vi "Boiler Controller.vi"(8 "error in":errorcluster, 9 "Controller Configuration":T1, 10 "Notifiers":T2, 11 "Message Queues":T3) -> (0 "error out":errorcluster)   [LabVIEW 2014, in "Controller.lvlib"]
uses:
  Controller.lvlib
  support/Message Queue/All Message Queues.ctl
  support/Message Queue/Message Cluster.ctl
  support/Notifiers/Notifiers.ctl
  Controller Configuration.ctl
  controls/MHL UI Data.ctl
  controls/MHL Status.ctl
  support/Boiler System Globals.vi
  <vilib>/Utility/error.llb/Error Cluster From Error Code.vi
  <vilib>/ErrorRing/Error Ring.xnode
  support/Message Queue/Message Queue.lvlib
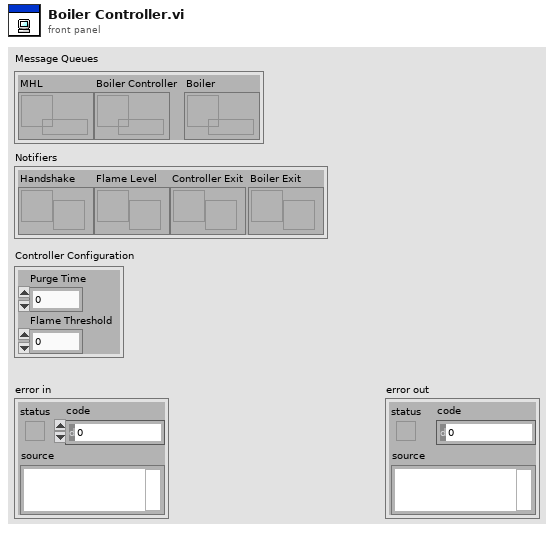
[diagram p1: front panel]
types:
  T1 = typedef "Controller.lvlib/Controller Configuration.ctl" = cluster{"Purge Time":u32, "Flame Threshold":u32}
  T2 = typedef "Notifiers.ctl" = cluster{"Handshake":refnum<notifier>, "Flame Level":refnum<notifier>, "Controller Exit":refnum<notifier>, "Boiler Exit":refnum<notifier>}
  T3 = typedef "Message Queue.lvlib/All Message Queues.ctl" = cluster{"MHL":refnum<queue>, "Boiler Controller":refnum<queue>, "Boiler":refnum<queue>}
  T4 = enum16{"open", "replace", "create", "open or create", "replace or create", "replace or create with confirmation"}
  T5 = typedef "MHL Status.ctl" = enum16{"Lockout", "Ready", "Pre-Purge", "Pre-Purge Complete", "Pilot On", "Boiler Running", "Shutdown", "Purge"}
  T6 = typedef "MHL UI Data.ctl" = cluster{"Status":string, "Fuel Control Valve":u32, "Primary Fan":bool, "Pilot Gas Valve":bool, "Pilot":bool, "Forced Draft Fan":bool, "MHL Status":T5}
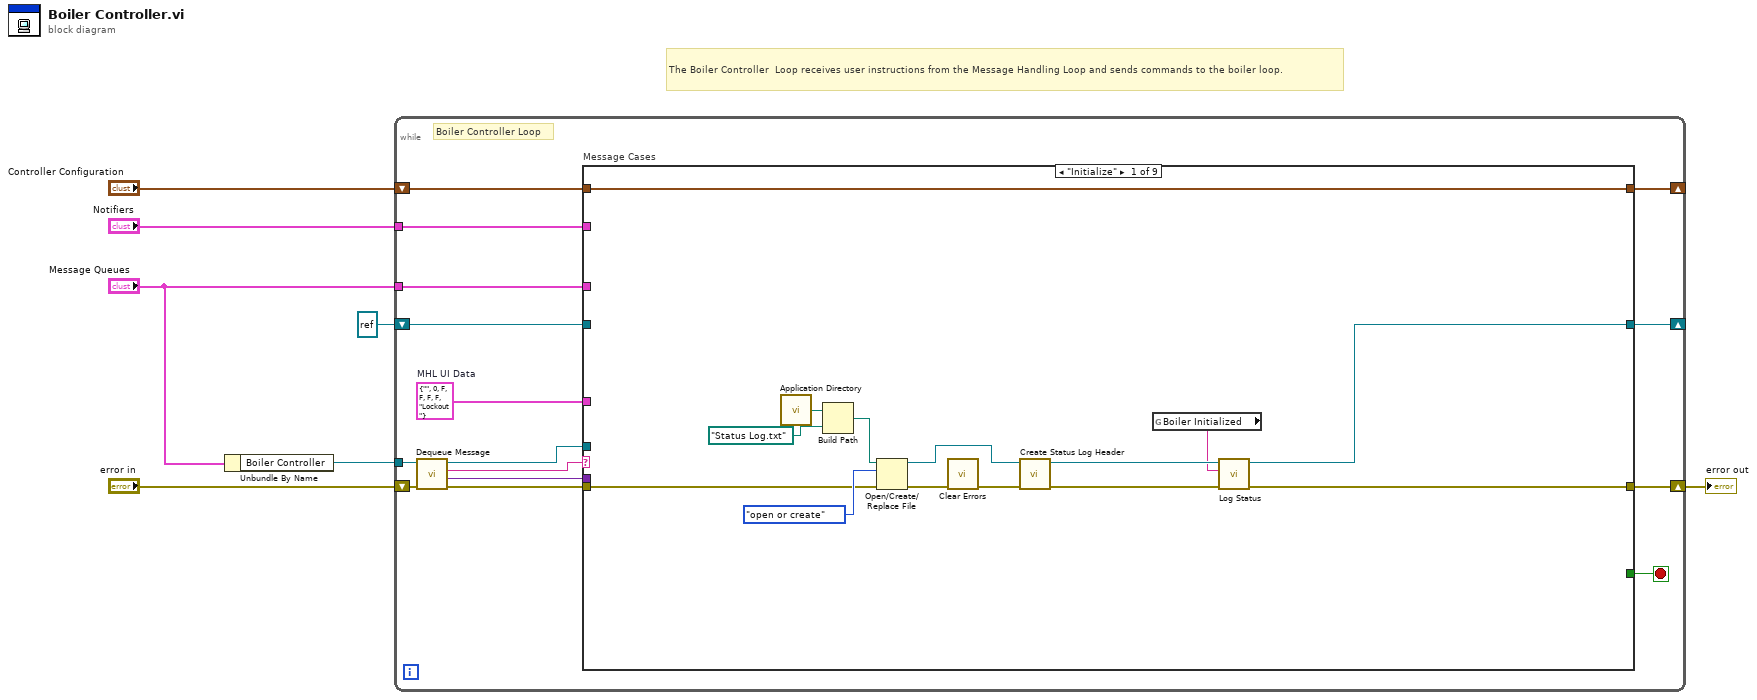
[diagram p0: block diagram]
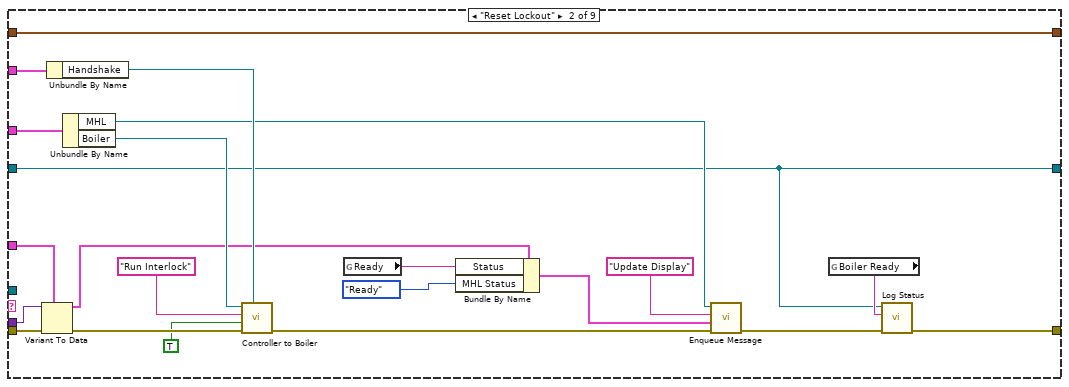
[diagram p2: hidden frame]
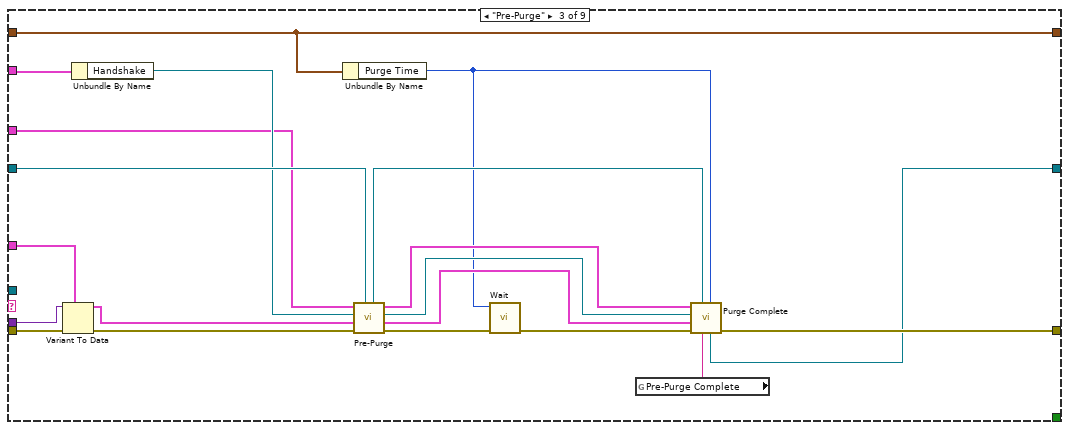
[diagram p3: hidden frame]
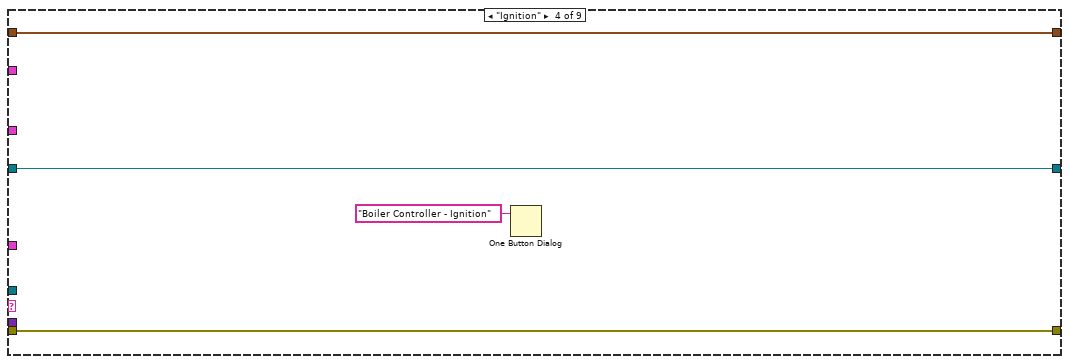
[diagram p4: hidden frame]
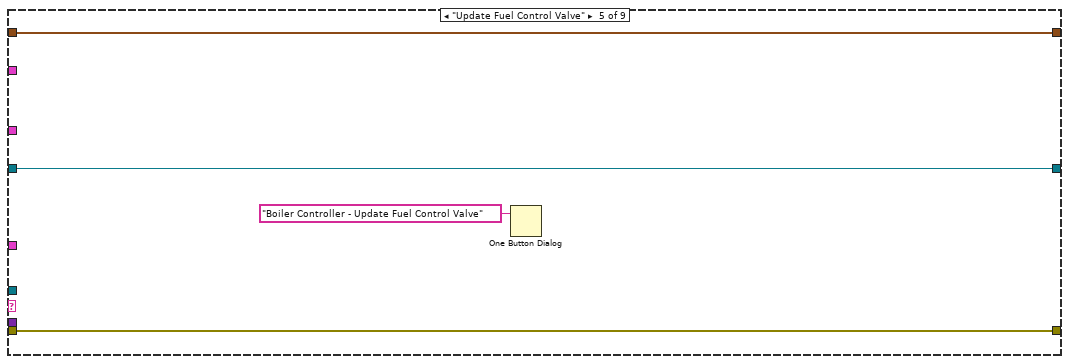
[diagram p5: hidden frame]
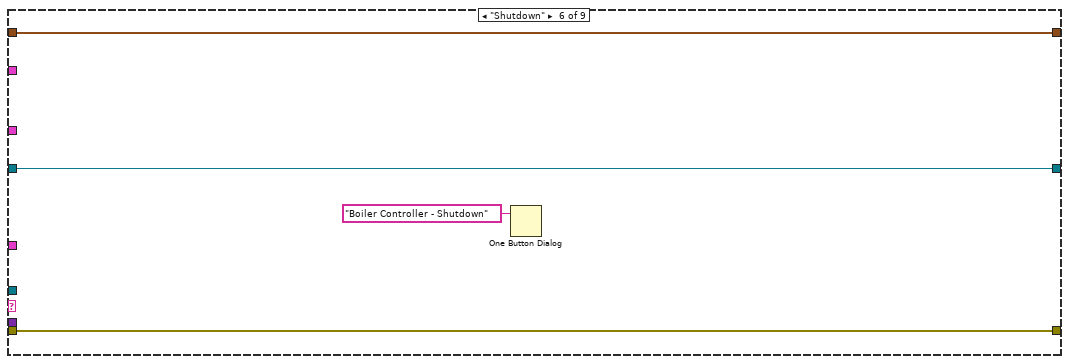
[diagram p6: hidden frame]
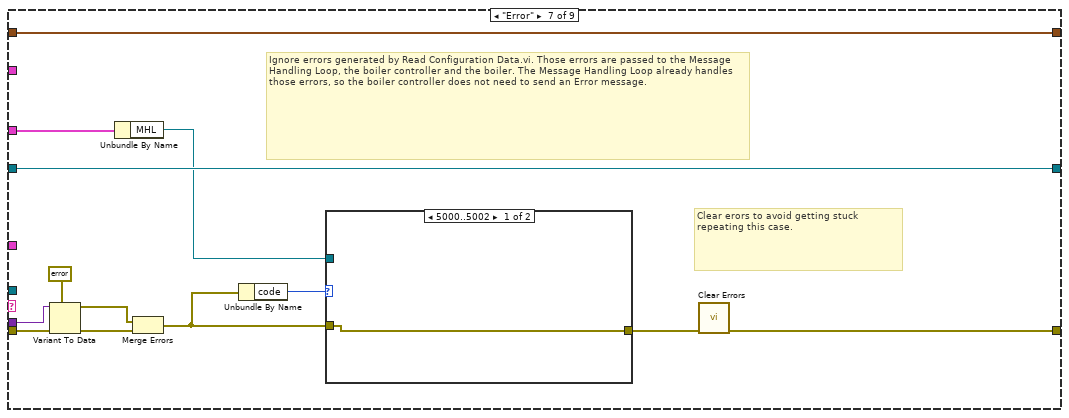
[diagram p7: hidden frame]
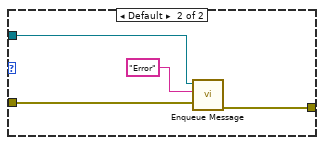
[diagram p8: hidden frame]
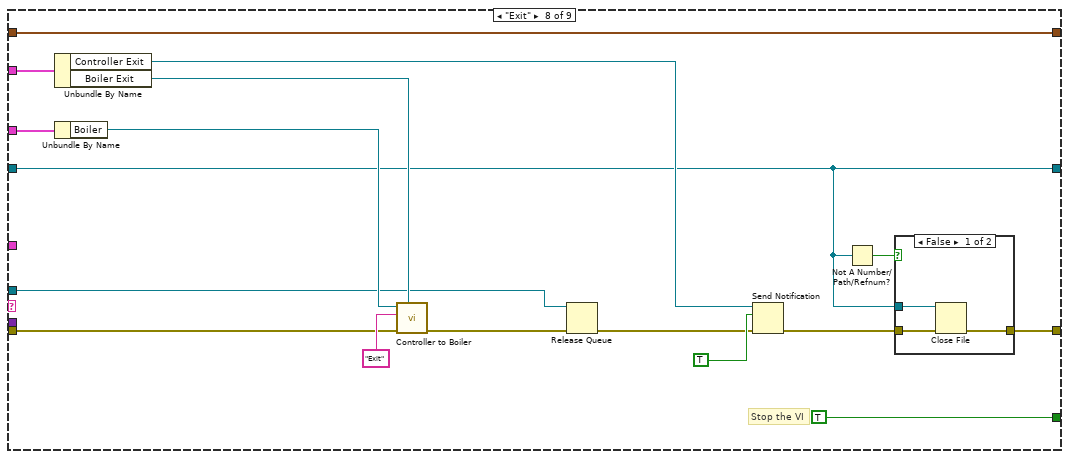
[diagram p9: hidden frame]
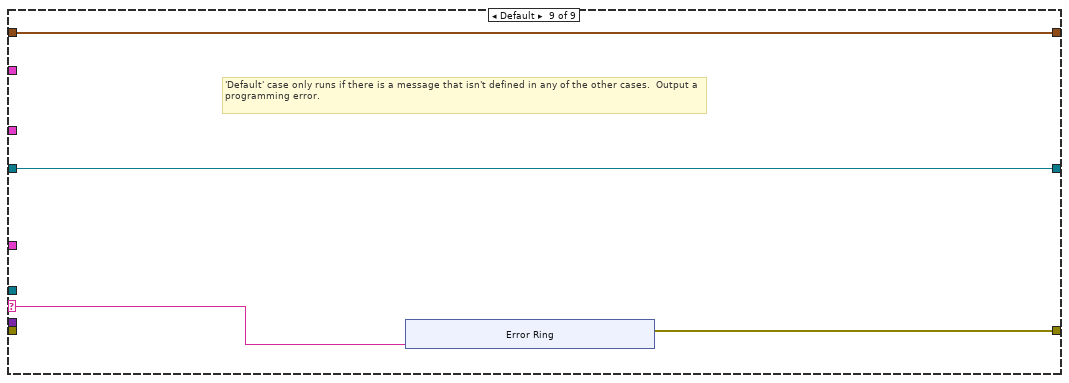
[diagram p11: hidden frame]
diagram:
  # "The Boiler Controller  Loop receives user instructions from the Message Handling Loop and sends commands to the boiler loop."
  n1 = Unbundle By Name("Message Queues") -> ("Boiler Controller"=w5:refnum<queue>)
  n2 = while {
    tunnel: w5 -> [w16]
    shift-right: [w15] -> w7
    shift-left: "error in" -> [w21]
    tunnel: "Message Queues" -> [w14]
    tunnel: "Notifiers" -> [w13]
    shift-right: [w12] -> _
    shift-left: refnum<file> refnum ("Log File Refnum out") -> [w11]
    shift-right: [w8] -> _
    shift-left: "Controller Configuration" -> [w9]
    stop <- w22 stop-if-true
    w10 = T6 {"Status"="", "Fuel Control Valve"=0, "Primary Fan"=FALSE, "Pilot Gas Valve"=FALSE, "Pilot"=FALSE, "Forced Draft Fan"=FALSE, "MHL Status"=enum."Lockout"}  # MHL UI Data
    # "Boiler Controller Loop"
    n3 = call "Dequeue Message.vi"("error in (no error)"=w21, "Message Queue"=w16) -> ("error out"=w20:errorcluster, "Message Data"=w18:variant, "Message"=w19:string, "dup Message Queue"=w17:refnum<queue>)  [unwired: 6 in]
    n4 = case "Message Cases" shown="\"Initialize\"" w19 {
      selector: w19 -> [_ _ _ _ _ _ _ _ w132]
      tunnel: w17 -> [_ _ _ _ _ _ _ w118 _]
      tunnel: w20 -> [w27 w58 w78 w82 w86 w90 w102 w117 _]
      tunnel: [w28 w54 w66 w82 w86 w90 w91 w110 w133] -> w15
      tunnel: [_ _ _ _ _ _ _ TRUE _] -> w22
      tunnel: w18 -> [_ w53 w76 _ _ _ w100 _ _]
      tunnel: w14 -> [_ w51 w70 _ _ _ w103 w115 _]
      tunnel: w13 -> [_ w49 w73 _ _ _ _ w114 _]
      tunnel: [w26 w39 w64 w80 w84 w88 w97 w109 w131] -> w12
      tunnel: w11 -> [_ w39 w72 w80 w84 w88 w97 w109 w131]
      tunnel: w10 -> [_ w52 w75 _ _ _ _ _ _]
      tunnel: w9 -> [w25 w37 w68 w79 w83 w87 w96 w113 w130]
      tunnel: [w25 w37 w68 w79 w83 w87 w96 w113 w130] -> w8
      frame "Initialize" {
        n5 = call <vilib>:"Application Directory.vi"() -> ("Application Directory"=w30:path)
        n6 = Build Path(base path=w30, name or relative path=path "Status Log.txt") -> (appended path=w33:path)
        n7 = Open/Create/Replace File(file path (use dialog)=w33, error in=w27, operation (0:open)=T4."open or create") -> (refnum out=w23:refnum<file>, error out=w31:errorcluster)  [unwired: 3 in, 1 out]
        n8 = call <vilib>:"Clear Errors.vi"("error in (no error)"=w31) -> ("error out"=w24:errorcluster)  [unwired: 5 in, 1 out]
        n9 = call "Create Status Log Header.vi"("error in"=w24, "Log File Refnum in"=w23) -> ("error out"=w36:errorcluster, "Log File Refnum out"=w35:refnum<file>)  [unwired: 8 in]
        n10 = global read "Boiler System Globals.vi" "Boiler Initialized"() -> (w34:string)
        n11 = call "Log Status.vi"("error in"=w36, "Event String"=w34, "Log File Refnum In"=w35) -> ("error out"=w28:errorcluster, "Log File Refnum Out"=w26:refnum<file>)  [unwired: 7 in]
      }
      frame "Reset Lockout" {
        n12 = Variant To Data(error in=w58, type=w52, Variant=w53) -> (data=w45:T6, error out=w57:errorcluster)
        n13 = Unbundle By Name(w49) -> ("Handshake"=w48:refnum<notifier>)
        n14 = Unbundle By Name(w51) -> ("MHL"=w41:refnum<queue>, "Boiler"=w50:refnum<queue>)
        n15 = call "Controller to Boiler.vi"("Notifier"=w48, "error in"=w57, "Message Data"=TRUE, "Message"="Run Interlock", "Boiler Queue in"=w50) -> ("error out"=w56:errorcluster)  [unwired: 4 in, 2 out]
        n16 = global read "Boiler System Globals.vi" "Ready"() -> (w44:string)
        n17 = Bundle By Name(cluster=w45, "Status"=w44, "MHL Status"=MHL_Status."Ready") -> (w43:T6)
        n18 = call "Enqueue Message.vi"("error in (no error)"=w56, "Message Data"=w43, "Message"="Update Display", "Message Queue"=w41) -> ("error out"=w55:errorcluster)  [unwired: 6 in, 1 out]
        n19 = global read "Boiler System Globals.vi" "Boiler Ready"() -> (w40:string)
        n20 = call "Log Status.vi"("error in"=w55, "Event String"=w40, "Log File Refnum In"=w39) -> ("error out"=w54:errorcluster)  [unwired: 7 in, 1 out]
      }
      frame "Pre-Purge" {
        n21 = Variant To Data(error in=w78, type=w75, Variant=w76) -> (data=w74:T6, error out=w77:errorcluster)
        n22 = Unbundle By Name(w73) -> ("Handshake"=w71:refnum<notifier>)
        n23 = Unbundle By Name(w68) -> ("Purge Time"=w60:u32)
        n24 = call "Pre-Purge.vi"("Log File Refnum in"=w72, "error in"=w77, "UI Data in"=w74, "Handshake Notifier in"=w71, "Message Queues in"=w70) -> ("error out"=w69:errorcluster, "UI Data out"=w63:T6, "Handshake Notifier out"=w62:refnum<notifier>, "Message Queues out"=w61:T3, "Log File Refnum out"=w65:refnum<file>)  [unwired: 2 in]
        n25 = call "Wait.vi"("error in"=w69, "Purge Time (s)"=w60) -> ("error out"=w67:errorcluster)  [unwired: 9 in]
        n26 = global read "Boiler System Globals.vi" "Pre-Purge Complete"() -> (w59:string)
        n27 = call "Purge Complete.vi"("Purge Time"=w60, "Status"=w59, "Log File Refnum in"=w65, "error in"=w67, "UI Data in"=w63, "Handshake Notifier in"=w62, "Message Queues in"=w61) -> ("error out"=w66:errorcluster, "Log File Refnum out"=w64:refnum<file>)  [unwired: 3 out]
      }
      frame "Ignition" {
        n28 = One Button Dialog(message="Boiler Controller - Ignition") -> ()  [unwired: 1 in, 1 out]
      }
      frame "Update Fuel Control Valve" {
        n29 = One Button Dialog(message="Boiler Controller - Update Fuel Control Valve") -> ()  [unwired: 1 in, 1 out]
      }
      frame "Shutdown" {
        n30 = One Button Dialog(message="Boiler Controller - Shutdown") -> ()  [unwired: 1 in, 1 out]
      }
      frame "Error" {
        # "Ignore errors generated by Read Configuration Data.vi. Those errors are passed to the Message Handling Loop, the boiler controller and the boiler. The Message Handling Loop already handles those errors, so the boiler controller does not need to send an Error message."
        # "Clear erors to avoid getting stuck repeating this case."
        n31 = Variant To Data(error in=w102, type=errorcluster {"status"=FALSE, "code"=0, "source"=""} ("error out"), Variant=w100) -> (data=w98:errorcluster, error out=w99:errorcluster)
        n32 = Unbundle By Name(w103) -> ("MHL"=w93:refnum<queue>)
        n33 = Merge Errors(w98, w99) -> (w92:errorcluster)
        n34 = Unbundle By Name(w92) -> ("code"=w95:i32)
        n35 = case shown="5000..5002" w95 {
          tunnel: w93 -> [_ w107]
          tunnel: [w104 w106] -> w94
          tunnel: w92 -> [w104 w105]
          frame 5000..5002 {
          }
          frame Default {
            n36 = call "Enqueue Message.vi"("Message Data"=w105, "Message"="Error", "Message Queue"=w107) -> ("error out"=w106:errorcluster)  [unwired: 7 in, 1 out]
          }
        }
        n37 = call <vilib>:"Clear Errors.vi"("error in (no error)"=w94) -> ("error out"=w91:errorcluster)  [unwired: 5 in, 1 out]
      }
      frame "Exit" {
        # "Stop the VI"
        n38 = Unbundle By Name(w114) -> ("Controller Exit"=w120:refnum<notifier>, "Boiler Exit"=w122:refnum<notifier>)
        n39 = Unbundle By Name(w115) -> ("Boiler"=w119:refnum<queue>)
        n40 = call "Controller to Boiler.vi"("Notifier"=w122, "error in"=w117, "Message"="Exit", "Boiler Queue in"=w119) -> ("error out"=w125:errorcluster)  [unwired: 5 in, 2 out]
        n41 = Release Queue(queue=w118, error in (no error)=w125) -> (error out=w121:errorcluster)  [unwired: 1 in, 2 out]
        n42 = Send Notification(notification=TRUE, notifier=w120, error in (no error)=w121) -> (error out=w111:errorcluster)  [unwired: 1 out]
        n43 = Not A Number/Path/Refnum?(number/path/refnum=w109) -> (NaN/Path/Refnum?=w112:bool)
        n44 = case shown="False" w112 {
          tunnel: [w127 w129] -> w110
          tunnel: w111 -> [w128 w129]
          tunnel: w109 -> [w126 _]
          frame False {
            n45 = Close File(refnum=w126, error in=w128) -> (error out=w127:errorcluster)  [unwired: 1 out]
          }
          frame True {
          }
        }
      }
      frame Default {
        # "'Default' case only runs if there is a message that isn't defined in any of the other cases.  Output a programming error."
        n46 = xnode "Error Ring"("parameter 0"=w132) -> ("error out"=w133:errorcluster)
      }
    }
  }
  "error out" <- w7
